vi "PH_Sequencer.PC CheckReadyShot.vi"(0 "i ref in":refnum<vi>, 5 "error in (no error)":errorcluster) -> (14 "i ref out":refnum<vi>, 19 "error out":errorcluster)   [LabVIEW 2014, in "PH_Sequencer.lvlib"]
doc: "This VI checks whether at least one device is selected and wether all subsystems are ready to shot. If so, it sets the GUI element and writes the information to own attributes."
uses:
  PH_Sequencer.lvlib
  PH_StatusHandler/PH_StatusHandler.Status.ctl
  PH_StatusHandler/PH_StatusHandler.lvlib
  PH_Common/PH_Common.lvlib
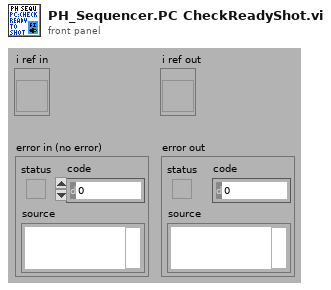
[diagram p1: front panel]
types:
  T1 = typedef "PH_Sequencer.lvlib/PH_Sequencer.i attribute.ctl" = cluster{"GUI Refs":cluster{"Main Off":refnum<vi>, "Fire":refnum<vi>, "Status":refnum<vi>, "Ready":refnum<vi>, "Waiting Time":refnum<vi>, "Timeout":refnum<vi>, "PPMA Ready":refnum<vi>, "Sequencer SM State":refnum<vi>, "PPPA Ready":refnum<vi>, "Calorimeter":refnum<vi>, "Beamline Ready":refnum<vi>, "Clear Beamline":refnum<vi>, "Linkage PPMA Rods":refnum<vi>, "Linkage Current PA":refnum<vi>, "Linkage Current MA":refnum<vi>, "Timing Ready":refnum<vi>, "State Timing":refnum<vi>, "Force Timing":refnum<vi>, "PSDB Shot Comment":refnum<vi>, "State PA Backreflection":refnum<vi>, "Beamline Z6 Ready":refnum<vi>, "Clear Z6 Beamline":refnum<vi>, "Sequence length":refnum<vi>, "Timing Mode":refnum<vi>, "Slow Trigger Settings":refnum<vi>, "Experiment Description":refnum<vi>, "State PSDB":refnum<vi>, "PSDB Ready":refnum<vi>, "Set PSDB Settings":refnum<vi>, "Get PSDB Info":refnum<vi>, "Take Snapshot":refnum<vi>, "Shottype":refnum<vi>, "Experiment":refnum<vi>, "Phase Frontends":refnum<vi>, "PP 45mm PILC in use":refnum<vi>}, "Status Info":cluster{"Machine Status":T2, "WaitingTime":i32, "Timeout":bool}, "Readyness":cluster{"Ready to shot":bool, "PPMA Ready":bool, "PPPA Ready":bool, "BL Ready":bool, "Timing Ready":bool, "BL Z6 Ready":bool, "PSDBReady":bool}, "Instancenames":cluster{"PPMA Rods":string, "PP Current Meas":string, "PH Beamline Chief":string, "PA Backrefl Meas":string, "Z6 Beamline Chief":string}, "Data to read":bool, "Calorimeter":cluster{"Instancename":string, "On":bool, "linked":bool}, "Linkage":cluster{"PPMA Rods":bool, "PP Current Meas":bool, "PHELIX Beamline Chief":bool, "PA Backrefl Meas":bool, "Z6 Beamline Chief":bool}, "Timing":cluster{"Instance":string, "linked":bool, "Status":T2, "Timing Mode":T3, "Slow Trigger Settings":T4, "Info available":cluster{"ext SlowTrigger":bool, "T2":bool, "Mode":bool, "Delay Slow Trigger":bool, "Phase FEs":bool}, "FE Phase":T5}, "Service ID R2S":i32, "PSDB":cluster{"Controller Instance":string, "Controller Status":T2, "Controller linked":bool, "Settings acknowledged":bool, "Current Experiment ID":i16, "Current Shot Type":i16, "Current Comment":string, "Remember Settings":bool, "Write 2 early":bool}, "PSDB Data":cluster{"Main Off?":bool, "Sequence Length":dbl, "Sequence startet":timestamp}, "6P 4Q Positions":cluster{"Instancename":string, "linked":bool, "Position":T6}[], "PUs":T7[]}
  T2 = typedef "PH_StatusHandler.lvlib/PH_StatusHandler.Status.ctl" = i16
  T3 = typedef "PH_Timing.lvlib/PH_Timing.Timing Mode.ctl" = cluster{"T2":i16, "Modeselector":enum32{"10 Hz", "0.5 Hz", "Shot"}}
  T4 = typedef "PH_Timing.lvlib/PH_Timing.Slow Trigger Settings.ctl" = cluster{"Delay":dbl, "externally triggered?":bool}
  T5 = typedef "PH_Timing.lvlib/PH_Timing.Phase FEs.ctl" = cluster{"Phase":dbl}
  T6 = typedef "PH_4_Pos_Selector.lvlib/PH_4_Pos_Selector.Position Selector.ctl" = u16
  T7 = typedef "PH_Sequencer.lvlib/PH_Sequencer.Head.ctl" = cluster{"PowerUnit":T8, "GUI Ref":refnum<vi>, "Information":T9, "linked?":bool, "GUI Ref Current Voltage":refnum<vi>}
  T8 = typedef "PH_PP_Common.lvlib/PH_PP_Common.PUs.ctl" = enum16{"no Info", "PA-19mm-1", "PA-19mm-2", "PA-45mm-PILC", "PA-45mm-MAIN", "MA-PU-1", "MA-PU-2", "MA-PU-3", "MA-PU-4", "MA-PU-5", "MA-PU-6", "MA-FR", "MA-PILC", "PA-45mm-DP"}
  T9 = typedef "PH_Sequencer.lvlib/PH_Sequencer.PU Information.ctl" = cluster{"State":T2, "Waiting Time [s]":dbl, "PU State SM":T10, "PU Timeout SM":T10}
  T10 = typedef "PH_PowerUnit_BaseClass.lvlib/PH_PowerUnit_BaseClass.SM States.ctl" = enum16{".", "Stand by", "Switch PU on", "Configure", "Set Default Voltage", "Set STANDBY", "Set READY", "Wait for Shot Cmd", "Open Dump Rods", "Open Ross Relais", "Close Ross Relais", "Switch PSU on", "Switch PSU off", "Charge", "Switch GD Channel on", "Close Dump Rods", "Rods-TO", "RR-TO", "PSU-TO", "Trigger-TO"}
  T11 = enum8{"Enabled", "Disabled", "Disabled and Grayed Out"}
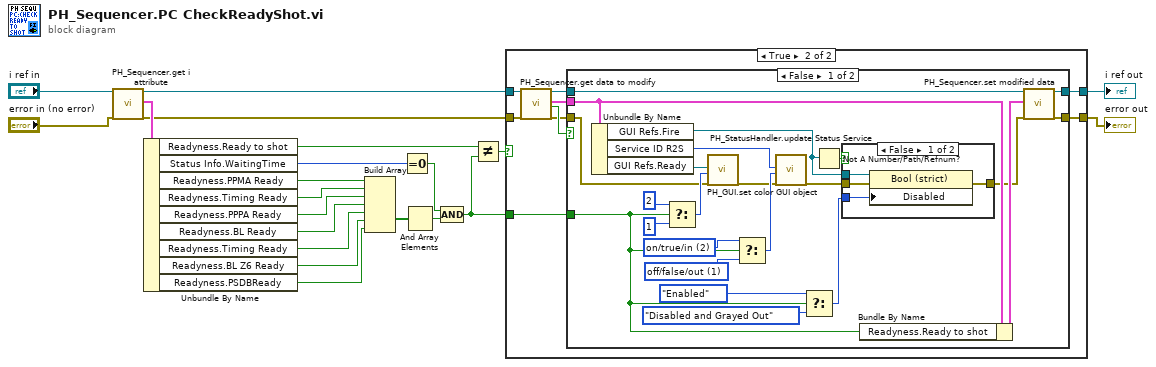
[diagram p0: block diagram]
diagram:
  n1 = call "PH_Sequencer.get i attribute.vi"("i ref in"="i ref in", "error in (no error)"="error in (no error)") -> ("i ref out"=w6:refnum<vi>, "i attribute"=w19:T1, "error out"=w4:errorcluster)  [unwired: 15 in]
  n2 = Unbundle By Name(w19) -> ("Readyness.Ready to shot"=w3:bool, "Status Info.WaitingTime"=w16:i32, "Readyness.PPMA Ready"=w18:bool, "Readyness.Timing Ready"=w14:bool, "Readyness.PPPA Ready"=w13:bool, "Readyness.BL Ready"=w11:bool, "Readyness.Timing Ready"=w10:bool, "Readyness.BL Z6 Ready"=w9:bool, "Readyness.PSDBReady"=w8:bool)
  n3 = Build Array(w18, w14, w13, w11, w10, w9, w8) -> (w17:bool[])
  n4 = Equal To 0?(x=w16) -> (x = 0?=w15:bool)
  n5 = And Array Elements(Boolean array=w17) -> (logical AND=w12:bool)
  n6 = Compound Arithmetic op=AND(w15, w12) -> (w2:bool)
  n7 = Not Equal?(x=w3, y=w2) -> (x != y?=w1:bool)
  n8 = case shown="True" w1 {
    tunnel: [w23 w31] -> w21
    tunnel: [w22 w29] -> w20
    tunnel: w6 -> [w23 w26]
    tunnel: w4 -> [w22 w25]
    tunnel: w2 -> [_ w24]
    frame False {
    }
    frame True {
      n9 = call "PH_Sequencer.get data to modify.vi"("i ref in"=w26, "error in (no error)"=w25) -> ("i ref out"=w30:refnum<vi>, "i attribute"=w27:T1, "timed out"=w32:bool, "error out"=w28:errorcluster)  [unwired: 14 in]
      n10 = case shown="False" w32 {
        tunnel: w27 -> [w52 _]
        tunnel: w28 -> [w38 w61]
        tunnel: [w55 w61] -> w29
        tunnel: w30 -> [w54 w62]
        tunnel: [w53 w62] -> w31
        tunnel: w24 -> [w35 _]
        frame False {
          w43 = T2 2 items=["no info", "off/false/out", "on/true/in", "Failure", "Alarm", "Status 1", "Status 2", "Status 3"] ("Status")
          w44 = T2 1 items=["no info", "off/false/out", "on/true/in", "Failure", "Alarm", "Status 1", "Status 2", "Status 3"] ("Status")
          n11 = Unbundle By Name(w52) -> ("GUI Refs.Fire"=w36:refnum<vi>, "Service ID R2S"=w46:i32, "GUI Refs.Ready"=w40:refnum<vi>)
          n12 = Select(t=2, s=w35, f=1) -> (s? t:f=w39:i32)
          n13 = call "PH_GUI.set color GUI object.vi"("GUI object Ref"=w40, "State"=w39, "error in (no error)"=w38) -> ("error out"=w37:errorcluster)  [unwired: 16 in]
          n14 = Select(t=w43, s=w35, f=w44) -> (s? t:f=w45:T2)
          n15 = call "PH_StatusHandler.update Status Service.vi"("Service ID"=w46, "Status"=w45, "error in (no error)"=w37) -> ("error out"=w47:errorcluster)  [unwired: 16 in]
          n16 = Select(t=T11."Enabled" ("Disabled"), s=w35, f=T11."Disabled and Grayed Out") -> (s? t:f=w49:T11)
          n17 = Not A Number/Path/Refnum?(number/path/refnum=w36) -> (NaN/Path/Refnum?=w50:bool)
          n18 = case shown="False" w50 {
            tunnel: w36 -> [w59 _]
            tunnel: w47 -> [w58 w60]
            tunnel: [w57 w60] -> w48
            tunnel: w49 -> [w56 _]
            frame False {
              n19 = property class="Bool (strict)"(reference=w59, error in=w58, "Disabled"=w56) -> (error out=w57:errorcluster)  [unwired: 1 out]
            }
            frame True {
            }
          }
          n20 = Bundle By Name(cluster=w52, "Readyness.Ready to shot"=w35) -> (w51:T1)
          n21 = call "PH_Sequencer.set modified data.vi"("i ref in"=w54, "i attribute"=w51, "error in (no error)"=w48) -> ("i ref out"=w53:refnum<vi>, "error out"=w55:errorcluster)  [unwired: 15 in]
        }
        frame True {
        }
      }
    }
  }
  "i ref out" <- w21
  "error out" <- w20
